vi "Experiment Executor.vi"(0 "Input Channels":string, 1 "Output Channels":string, 2 "Output Waveforms":waveform(dbl)[](array[waveform])) -> ()   [LabVIEW 2013]
doc: "Run and experiment by forcing the given output waveforms onto the desired output channels, while reading data from the input channels provided. Once the input data is ready, it is dimensioned and saved in a functional global variable."
uses:
  <vilib>/DAQmx/write.llb/DAQmx Write (Analog 1D Wfm NChan NSamp).vi
  <vilib>/DAQmx/read.llb/DAQmx Read (Analog 2D DBL NChan NSamp).vi
  <vilib>/DAQmx/create/channels.llb/DAQmx Create Channel (AO-Voltage-Basic).vi
  <vilib>/DAQmx/configure/timing.llb/DAQmx Timing (Use Waveform).vi
  <vilib>/DAQmx/configure/trigger.llb/DAQmx Start Trigger (Digital Edge).vi
  <vilib>/DAQmx/create/channels.llb/DAQmx Create Channel (AI-Voltage-Basic).vi
  <vilib>/DAQmx/configure/timing.llb/DAQmx Timing (Sample Clock).vi
  <vilib>/DAQmx/miscellaneous.llb/DAQmx Fill In Error Info.vi
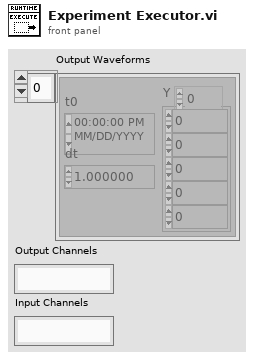
[diagram p1: front panel]
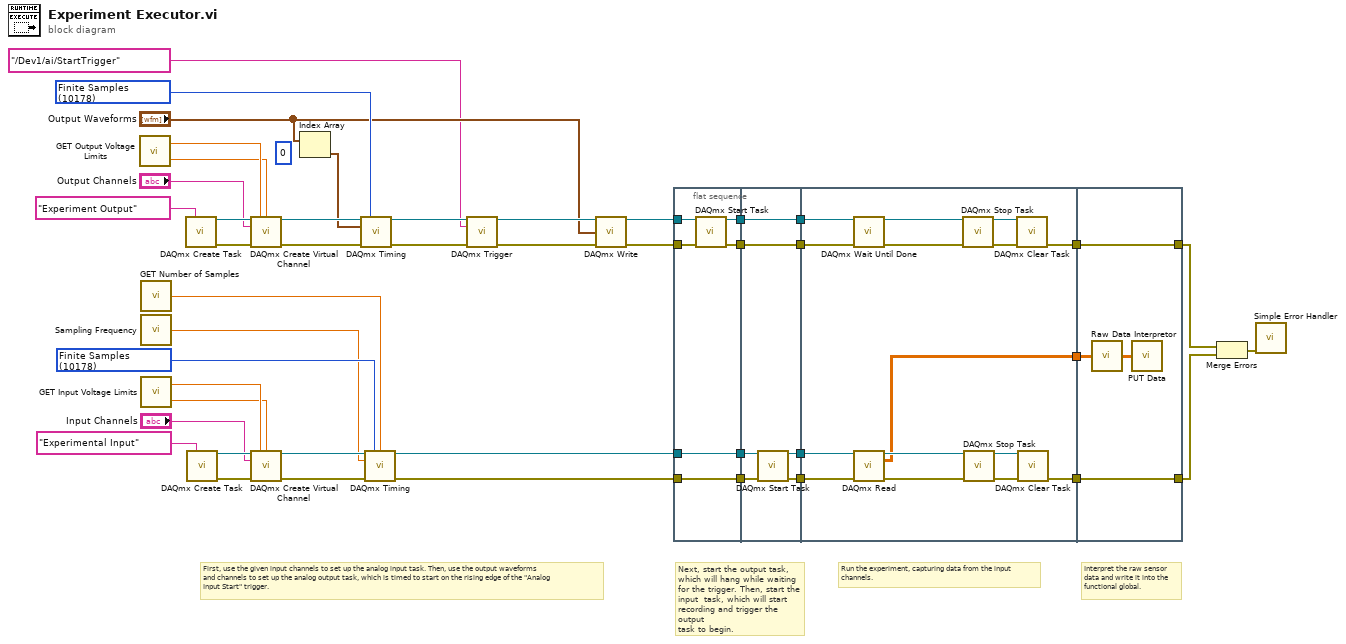
[diagram p0: block diagram]
diagram:
  w13 = 10178 items=["Finite Samples"=10178, "Continuous Samples"=10123, "Hardware Timed Single Point"=12522] ("sample mode")
  (unwired) 0 ("index")
  w29 = 10178 items=["Finite Samples"=10178, "Continuous Samples"=10123, "Hardware Timed Single Point"=12522] ("sample mode")
  # "Interpret the raw sensor\ndata and write it into the\nfunctional global."
  # "Run the experiment, capturing data from the input \nchannels."
  # "Next, start the output task,\nwhich will hang while waiting\nfor the trigger. Then, start the\ninput  task, which will start \nrecording and trigger the output\ntask to begin."
  # "First, use the given input channels to set up the analog input task. Then, use the output waveforms\nand channels to set up the analog output task, which is timed to start on the rising edge of the \"Analog\nInput Start\" trigger."
  n1 = call "GET Output Voltage Limits.vi"() -> ("Minimum Output Voltage"=w6:dbl, "Maximum Output Voltage"=w7:dbl)  [unwired: 2 in]
  n2 = call "GET Number of Samples.vi"() -> ("Number of Samples"=w12:dbl)
  n3 = call "Sampling Frequency.vi"() -> ("Sampling Frequency"=w11:dbl)
  n4 = call "GET Input Voltage Limits.vi"() -> ("Minimum Input Voltage"=w8:dbl, "Maximum Input Voltage"=w9:dbl)  [unwired: 2 in]
  n5 = call <vilib>:"DAQmx Create Task.vi"("new task name"="Experiment Output") -> ("task out"=w39:refnum<k21>, "error out"=w45:errorcluster)  [unwired: 13 in]
  n6 = call <vilib>:"DAQmx Create Task.vi"("new task name"="Experimental Input") -> ("task out"=w25:refnum<k21>, "error out"=w24:errorcluster)  [unwired: 13 in]
  n7 = call-poly <vilib>:"DAQmx Create Virtual Channel.vi"("task in"=w39, "maximum value"=w7, "minimum value"=w6, "physical channels"="Output Channels", "error in"=w45) -> ("task out"=w38:refnum<k21>, "error out"=w44:errorcluster)  [unwired: 9 in]
  n8 = call-poly <vilib>:"DAQmx Create Virtual Channel.vi"("task in"=w25, "maximum value"=w9, "minimum value"=w8, "physical channels"="Input Channels", "error in"=w24) -> ("task out"=w23:refnum<k21>, "error out"=w22:errorcluster)  [unwired: 9 in]
  n9 = Index Array(array="Output Waveforms") -> (element=w28:waveform(dbl))  [unwired: 1 in]
  n10 = call-poly <vilib>:"DAQmx Timing.vi"("task/channels in"=w38, "sample mode"=w29, "waveform"=w28, "error in"=w44) -> ("task out"=w37:refnum<k21>, "error out"=w43:errorcluster)  [unwired: 10 in]
  n11 = call-poly <vilib>:"DAQmx Timing.vi"("task/channels in"=w23, "sample mode"=w13, "samples per channel"=w12, "rate"=w11, "error in"=w22) -> ("task out"=w20:refnum<k21>, "error out"=w18:errorcluster)  [unwired: 9 in]
  n12 = call-poly <vilib>:"DAQmx Trigger.vi"("task/channels in"=w37, "source"=tag "/Dev1/ai/StartTrigger" ("DAQmx Terminal"), "error in"=w43) -> ("task out"=w36:refnum<k21>, "error out"=w42:errorcluster)  [unwired: 11 in]
  n13 = call-poly <vilib>:"DAQmx Write.vi"("task/channels in"=w36, "data"="Output Waveforms", "error in"=w42) -> ("task out"=w40:refnum<k21>, "error out"=w41:errorcluster)  [unwired: 10 in, 1 out]
  n14 = flat-sequence {
    tunnel: w41 -> [w51]
    tunnel: w40 -> [w49]
    tunnel: [w50] -> w35
    tunnel: [w48] -> w33
    tunnel: [w47] -> w21
    tunnel: w20 -> [w47]
    tunnel: [w46] -> w19
    tunnel: w18 -> [w46]
    tunnel: w35 -> [w57]
    tunnel: [w57] -> w34
    tunnel: w33 -> [w56]
    tunnel: [w56] -> w32
    tunnel: w21 -> [w55]
    tunnel: w19 -> [w54]
    tunnel: [w53] -> w17
    tunnel: [w52] -> w16
    tunnel: w34 -> [w72]
    tunnel: w32 -> [w71]
    tunnel: w17 -> [w66]
    tunnel: w16 -> [w65]
    tunnel: [w60] -> w5
    tunnel: [w59] -> w4
    tunnel: [w58] -> w2
    tunnel: w5 -> [w75]
    tunnel: [w74] -> w3
    tunnel: w4 -> [w74]
    tunnel: [w73] -> w1
    tunnel: w2 -> [w73]
    frame #0 {
      n15 = call <vilib>:"DAQmx Start Task.vi"("task/channels in"=w49, "error in"=w51) -> ("task out"=w48:refnum<k21>, "error out"=w50:errorcluster)  [unwired: 12 in]
    }
    frame #1 {
      n16 = call <vilib>:"DAQmx Start Task.vi"("task/channels in"=w55, "error in"=w54) -> ("task out"=w53:refnum<k21>, "error out"=w52:errorcluster)  [unwired: 12 in]
    }
    frame #2 {
      n17 = call <vilib>:"DAQmx Wait Until Done.vi"("task/channels in"=w71, "error in"=w72) -> ("task out"=w70:refnum<k21>, "error out"=w69:errorcluster)  [unwired: 12 in]
      n18 = call-poly <vilib>:"DAQmx Read.vi"("task/channels in"=w66, "error in"=w65) -> ("task out"=w64:refnum<k21>, "data"=w60:dbl[][], "error out"=w63:errorcluster)  [unwired: 11 in]
      n19 = call <vilib>:"DAQmx Stop Task.vi"("task/channels in"=w70, "error in"=w69) -> ("task out"=w67:refnum<k21>, "error out"=w68:errorcluster)  [unwired: 12 in]
      n20 = call <vilib>:"DAQmx Stop Task.vi"("task/channels in"=w64, "error in"=w63) -> ("task out"=w62:refnum<k21>, "error out"=w61:errorcluster)  [unwired: 12 in]
      n21 = call <vilib>:"DAQmx Clear Task.vi"("task in"=w67, "error in"=w68) -> ("error out"=w58:errorcluster)  [unwired: 13 in]
      n22 = call <vilib>:"DAQmx Clear Task.vi"("task in"=w62, "error in"=w61) -> ("error out"=w59:errorcluster)  [unwired: 13 in]
    }
    frame #3 {
      n23 = call "Raw Data Interpretor.vi"("Sensor Data"=w75) -> ("Interpreted Data"=w76:dbl[][])
      n24 = call "PUT Data.vi"("Data"=w76) -> ()
    }
  }
  n25 = Merge Errors(w1, w3) -> (w10:errorcluster)
  n26 = call <vilib>:"Simple Error Handler.vi"("error in (no error)"=w10) -> ()  [unwired: 4 in, 5 out]
